vi "subEvent.vi"(8 "error in (no error)":errorcluster, 11 "SalProcess in":refnum<class "SalProcess.lvclass">) -> (0 "error out":errorcluster, 1 "function return":i32, 2 "variant":variant, 3 "SalProcess out":refnum<class "SalProcess.lvclass">)   [LabVIEW 2018, in "SalProcess.lvclass"]
doc: "Subscribe the event."
uses:
  SalProcess.lvclass
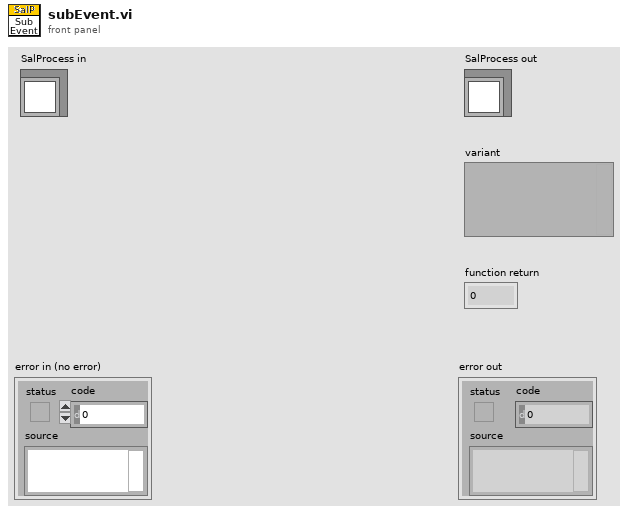
[diagram p1: front panel]
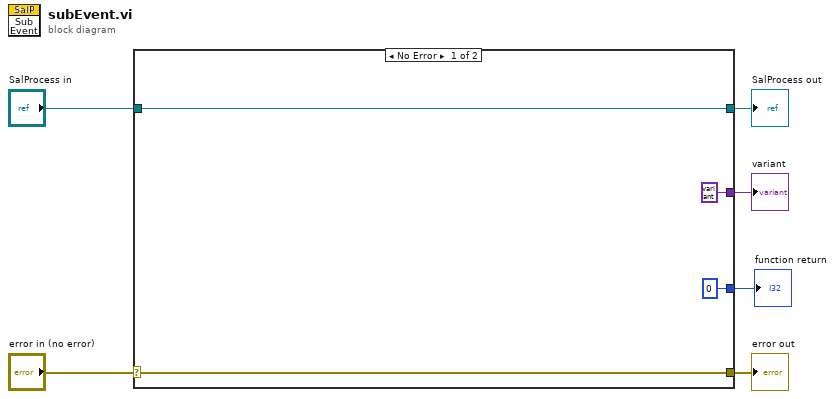
[diagram p0: block diagram]
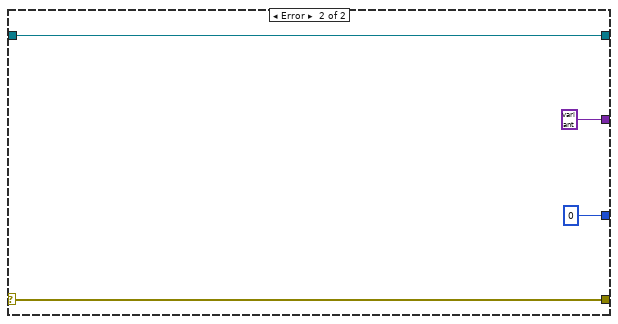
[diagram p2: hidden frame]
diagram:
  n1 = case shown="No Error" "error in (no error)" {
    selector: "error in (no error)" -> [w10 w14]
    tunnel: [w10 w14] -> w5
    tunnel: [w9 w13] -> w3
    tunnel: "SalProcess in" -> [w9 w13]
    tunnel: [variant ("variant") variant ("variant")] -> w2
    tunnel: [0 ("function return") 0 ("function return")] -> w1
    frame No Error {
    }
    frame Error {
    }
  }
  "error out" <- w5
  "SalProcess out" <- w3
  "function return" <- w1
  "variant" <- w2
